vi "通知.vi"() -> ()   [LabVIEW 2020]
panel:
  in  "颜色盒":u32(colorbox)
  in  "Reset":bool
  in  "Time":dbl=2.0 format="%#_13g"
  out "字符串":string
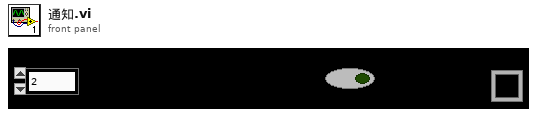
[diagram p1: front panel]
types:
  T1 = typedef "LVRectTypeDef.ctl" = cluster{"Left":i16, "Top":i16, "Right":i16, "Bottom":i16}
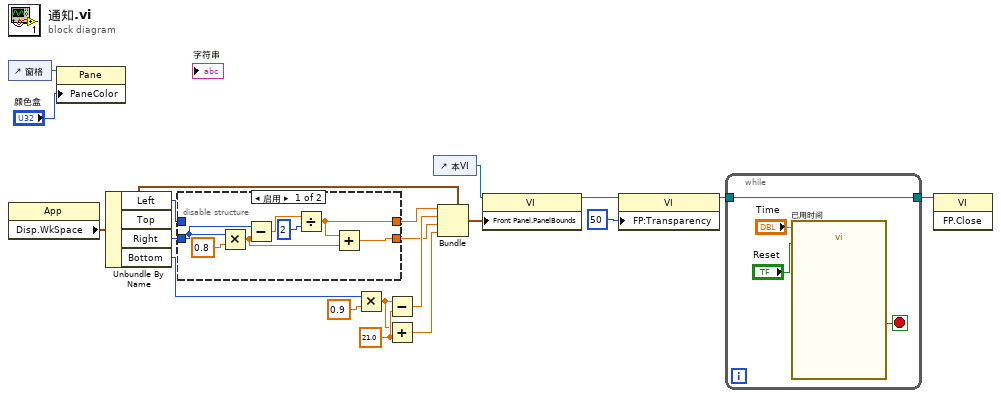
[diagram p0: block diagram]
diagram:
  w12 = 21.0 ("y")
  n1 = control-ref of="窗格"() -> (w18:refnum<vi>)
  n2 = property class="App"() -> ("Disp.WkSpace"=w8:T1)  [unwired: 2 in, 2 out]
  n3 = property class="Pane"(reference=w18, "PaneColor"="颜色盒") -> ()  [unwired: 1 in, 2 out]
  n4 = Unbundle By Name(w8) -> ("Left"=w1:i16, "Right"=w3:i16, "Bottom"=w7:i16)  [unwired: 1 out]
  n5 = disable-structure shown="启用" {
    disable-tunnel: [w26 w27] -> w6
    disable-tunnel: [w25 w28] -> w5
    disable-tunnel: w3 -> [w22 w27]
    disable-tunnel: w1 -> [_ w28]
    frame Enabled {
      n6 = Multiply(x=w22, y=0.8) -> (x*y=w20:dbl)
      n7 = Subtract(x=w22, y=w20) -> (x-y=w23:dbl)
      n8 = Divide(x=w23, y=i16 2) -> (x/y=w25:dbl)
      n9 = Add(x=w25, y=w20) -> (x+y=w26:dbl)
    }
    frame Disabled {
    }
  }
  n10 = Multiply(x=w7, y=0.9) -> (x*y=w11:dbl)
  n11 = Subtract(x=w11, y=w12) -> (x-y=w13:dbl)
  n12 = Add(x=w11, y=w12) -> (x+y=w14:dbl)
  n13 = control-ref of="本VI"() -> (w4:refnum<vi>)
  n14 = Bundle(cluster=w8, "Left"=w5, "Top"=w13, "Right"=w6, "Bottom"=w14) -> (w9:T1)
  n15 = property class="VI"(reference=w4, "Front Panel.PanelBounds"=w9) -> (reference out=w15:refnum<vi>)  [unwired: 1 in, 1 out]
  n16 = property class="VI"(reference=w15, "FP:Transparency"=u8 50 ("前面板窗口:透明度")) -> (reference out=w2:refnum<vi>)  [unwired: 1 in, 1 out]
  n17 = while {
    tunnel: [w29] -> w19
    tunnel: w2 -> [w29]
    stop <- w32 stop-if-true
    n18 = call "已用时间"("Time Target (s)"="Time", "Reset"="Reset") -> ("Time has Elapsed"=w32:bool)  [unwired: 10 in, 7 out]
  }
  n19 = invoke class="VI" method="FP.Close"(reference=w19) -> ()  [unwired: 2 in, 3 out]
